vi "Axis Image Stream Get.vi"(10 "Acquire Params":T1={"fps"=10, "Compression"=30, "X"=320, "Y"=240, "Enable Color?"=TRUE, "Rotation"=enum."0"}, 11 "IP Address":string="192.168.1.101") -> (3 "Raw Image Data":string)   [LabVIEW 2017]
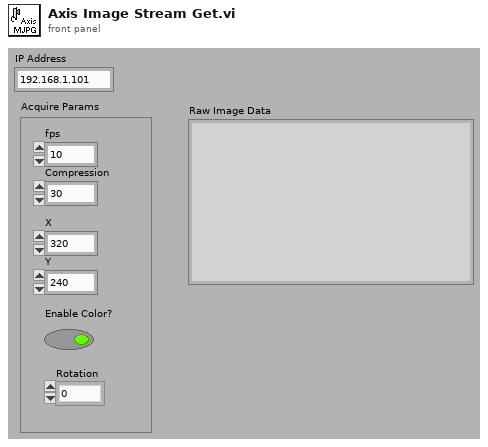
[diagram p1: front panel]
types:
  T1 = cluster{"fps":i32, "Compression":i32, "X":i32, "Y":i32, "Enable Color?":bool, "Rotation":enum16{"0", "90", "180", "270"}}
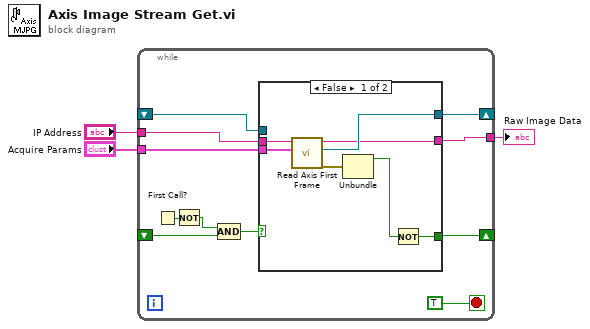
[diagram p0: block diagram]
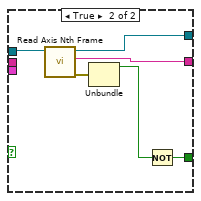
[diagram p2: hidden frame]
diagram:
  n1 = while {
    tunnel: "Acquire Params" -> [w14]
    tunnel: "IP Address" -> [w13]
    shift-right: [w11] -> _
    shift-left: _ -> [w12]
    shift-right: [w9] -> _
    shift-left: _ -> [w10]
    tunnel: [w8] -> w1
    stop <- TRUE stop-if-true
    n2 = First Call?() -> (First Call?: T/F=w5:bool)
    n3 = Not(x=w5) -> (.not. x?=w4:bool)
    n4 = Compound Arithmetic op=AND(w4, w12) -> (w6:bool)
    n5 = case shown="False" w6 {
      tunnel: w14 -> [w21 _]
      tunnel: w13 -> [w20 _]
      tunnel: [w17 w25] -> w11
      tunnel: w10 -> [_ w23]
      tunnel: [w16 w24] -> w9
      tunnel: [w15 w22] -> w8
      frame False {
        n6 = call <vilib>:"Read Axis First Frame.vi"("Acquire Params"=w21, "address"=w20) -> ("error out"=w19:errorcluster, "connection ID out"=w16:refnum<k5>, "Raw Image Data"=w15:string)  [unwired: 7 in]
        n7 = Unbundle(w19) -> ("status"=w18:bool)  [unwired: 2 out]
        n8 = Not(x=w18) -> (.not. x?=w17:bool)
      }
      frame True {
        n9 = call <vilib>:"Read Axis Nth Frame.vi"("connection ID"=w23) -> ("error out"=w26:errorcluster, "Raw Image Data"=w22:string, "connection ID out"=w24:refnum<k5>)  [unwired: 8 in]
        n10 = Unbundle(w26) -> ("status"=w27:bool)  [unwired: 2 out]
        n11 = Not(x=w27) -> (.not. x?=w25:bool)
      }
    }
  }
  "Raw Image Data" <- w1
